vi "Encoding Message from GUI.vi"(8 "Data":string, 9 "Message":string, 10 "uS/GD ID":string, 11 "uService Template in":refnum<class "TCP Text Writer.lvclass">) -> (2 "Variant":variant, 3 "uService Template out":refnum<class "TCP Text Writer.lvclass">)   [LabVIEW 2026, in "TALOS.lvlib" / "TCP Text Writer.lvlib" / "TCP Text Writer.lvclass"]
uses:
  TCP Text Writer.lvclass
  Support VIs/Global Constants.vi
  TALOS.lvlib
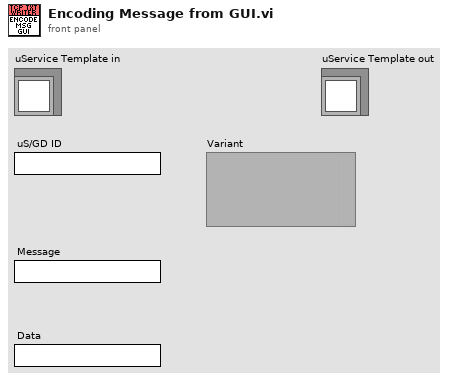
[diagram p1: front panel]
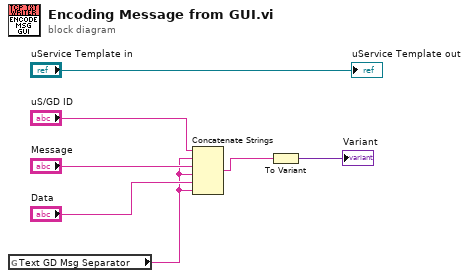
[diagram p0: block diagram]
diagram:
  n1 = global read "Global Constants.vi" "Text GD Msg Separator"() -> (w3:string)
  n2 = Concatenate Strings("uS/GD ID", w3, "Message", w3, "Data", w3) -> (w2:string)
  n3 = To Variant(anything=w2) -> (Variant=→"Variant":variant)
  "uService Template out" <- "uService Template in"
